vi "XML Parse DBL-Array.vi"(3 "Attribut Name":string[](array[string]), 7 "XML Response":string) -> (0 "Werte (DBL)":dbl[](array[numeric]), 2 "XML Response gekürzt":string)   [LabVIEW 2020, in "FT-IR.lvlib" / "TOOLweb Interface.lvlib" / "TOOLweb Interface Hilfs-VIs.lvlib"]
doc: "Sucht in dem XML-Poll-Response-String \"XML-Response\" alle Einträge mit den Elementnamen im Array \"Attribut Name\" und liefert deren Werte im DBL-Array \"Werte (DBL)\". \n\nDer Eintrag wird dann entfernt, damit eine weiteres Parser-VI am Ausgang \"XML Response gekürzt\" nicht wieder den ganzen String durchsuchen muss."
uses:
  TOOLweb Interface Hilfs-VIs.lvlib
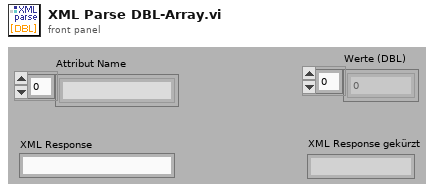
[diagram p1: front panel]
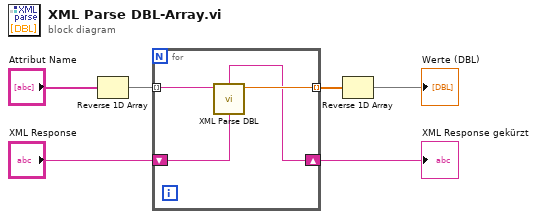
[diagram p0: block diagram]
diagram:
  n1 = Reverse 1D Array(array="Attribut Name") -> (reversed array=w3:string[])
  n2 = for {
    tunnel: w3 -> [w10] mode=indexing
    shift-right: [w7] -> w5
    shift-left: "XML Response" -> [w9]
    tunnel: [w8] -> w2 mode=indexing
    n3 = call "XML Parse DBL.vi"("Attribut Name"=w10, "XML Response"=w9) -> ("Wert (DBL)"=w8:dbl, "XML Response gekürzt"=w7:string)  [unwired: 6 out]
  }
  "XML Response gekürzt" <- w5
  n4 = Reverse 1D Array(array=w2) -> (reversed array=→"Werte (DBL)":dbl[])
